vi "Set Initialization Data - DataSave Worker.vi"(8 "error in":errorcluster, 11 "DAQ Worker in":refnum<class "DAQ Worker.lvclass">) -> (0 "error out":errorcluster, 3 "DAQ Worker out":refnum<class "DAQ Worker.lvclass">)   [LabVIEW 2020, in "DAQ Worker.lvclass"]
doc: "In this VI you can set the initialization data of a statically-linked subWorker."
uses:
  DAQ Worker.lvclass
  DataSave Worker/Initialization Data.ctl
  DataSave Worker/Response Cases.ctl
  DAQ Worker.lvclass/DAQ Worker.ctl
  DataSave Worker/DataSave Worker.lvclass
  C:/Program Files (x86)/National Instruments/LabVIEW 2020/vi.lib/addons/_Workers/Library/Classes/Worker/Worker.lvclass
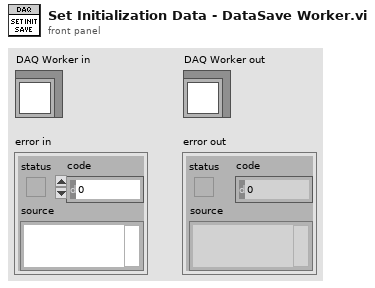
[diagram p1: front panel]
types:
  T1 = typedef "DataSave Worker.lvclass/Initialization Data.ctl" = cluster{"Response Cases":T2}
  T2 = typedef "DataSave Worker.lvclass/Response Cases.ctl" = cluster{"Placeholder - Can be deleted":string}
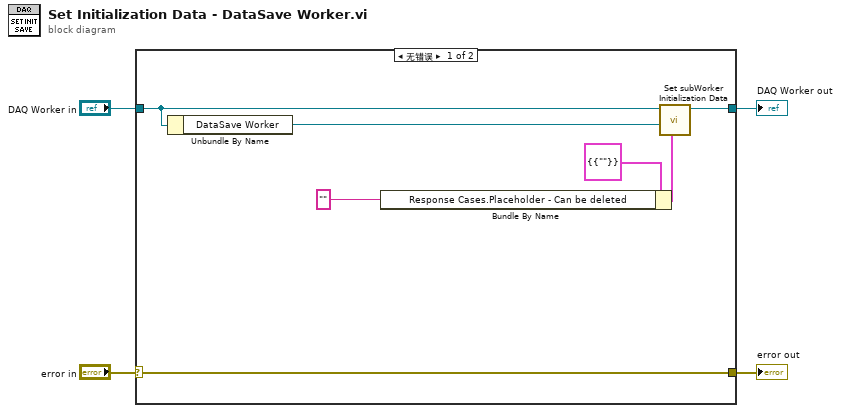
[diagram p0: block diagram]
diagram:
  n1 = case shown="无错误" "error in" {
    selector: "error in" -> [w11 w13]
    tunnel: [w11 w13] -> w3
    tunnel: [w9 w12] -> w2
    tunnel: "DAQ Worker in" -> [w8 w12]
    frame No Error {
      n2 = Unbundle By Name(w8) -> ("DataSave Worker"=w10:refnum<class "DataSave Worker.lvclass">)
      n3 = Bundle By Name(cluster=T1 {"Response Cases"={"Placeholder - Can be deleted"=""}} ("Initialization Data"), "Response Cases.Placeholder - Can be deleted"="" ("Placeholder")) -> (w6:T1)
      n4 = call-dynamic "Set subWorker Initialization Data.vi"("Initialization Data"=w6, "subWorker"=w10, "Worker"=w8) -> ("Worker out"=w9:refnum<class "DAQ Worker.lvclass">)  [unwired: 8 in]
    }
    frame Error {
    }
  }
  "error out" <- w3
  "DAQ Worker out" <- w2
